vi "Global Shtop.vi"() -> ()   [LabVIEW 2016]
panel:
  in  "SHTOP":bool
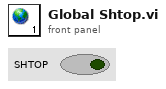
[diagram p1: front panel]
diagram:
